vi "Main.vi"(8 "error in":errorcluster, 11 "Head Worker in":refnum<class "Head Worker.lvclass">) -> (0 "error out":errorcluster, 3 "Head Worker out":refnum<class "Head Worker.lvclass">)   [LabVIEW 2017, in "Head Worker.lvclass"]
doc: "The <b>Queued Message Handler</b> of the Worker that owns this VI."
uses:
  Head Worker.lvclass
  Head Worker.lvclass/Head Worker.ctl
  Initialization Data.ctl
  Response Cases.ctl
  Main UI/Main UI.lvclass
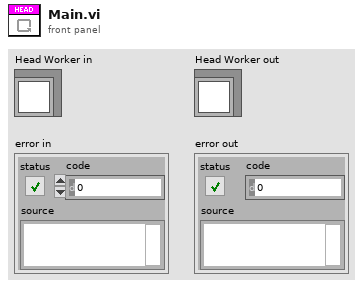
[diagram p1: front panel]
types:
  T1 = typedef "Head Worker.lvclass/Initialization Data.ctl" = cluster{"Response Cases":T2}
  T2 = typedef "Head Worker.lvclass/Response Cases.ctl" = cluster{"Placeholder - Can be deleted":string}
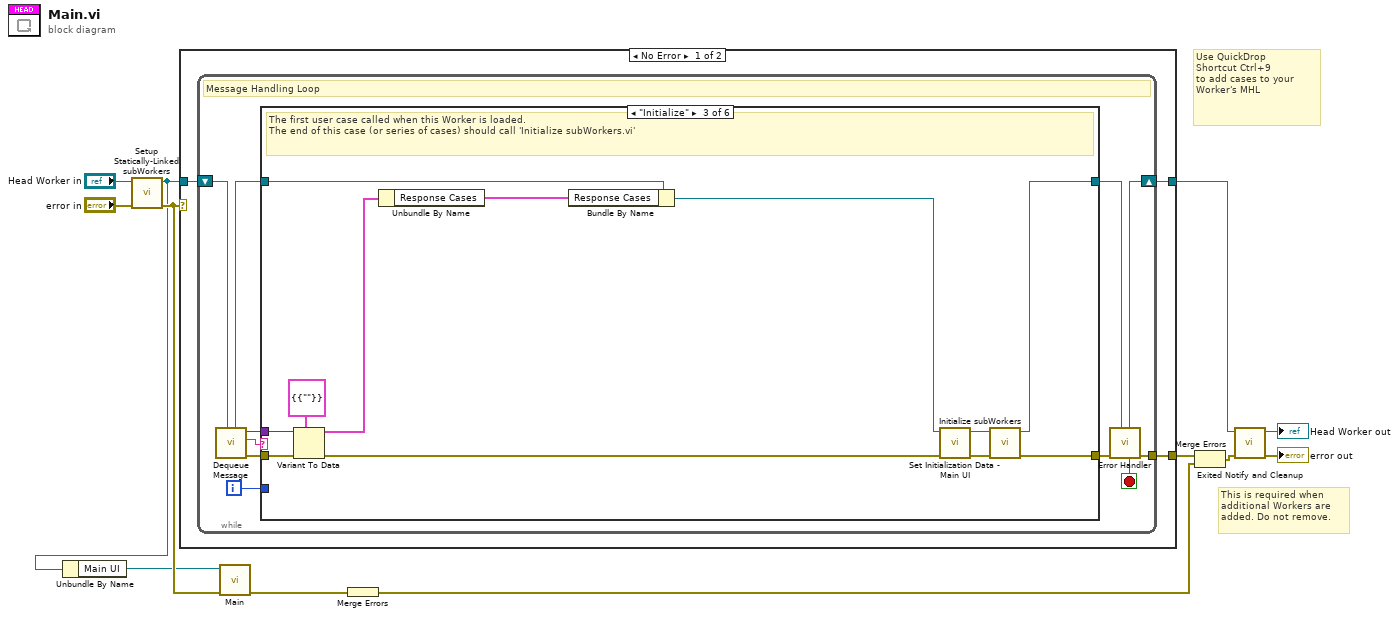
[diagram p0: block diagram]
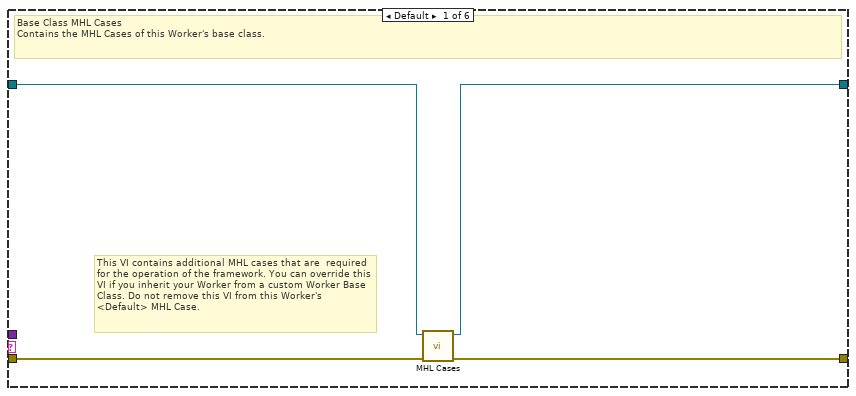
[diagram p2: hidden frame]
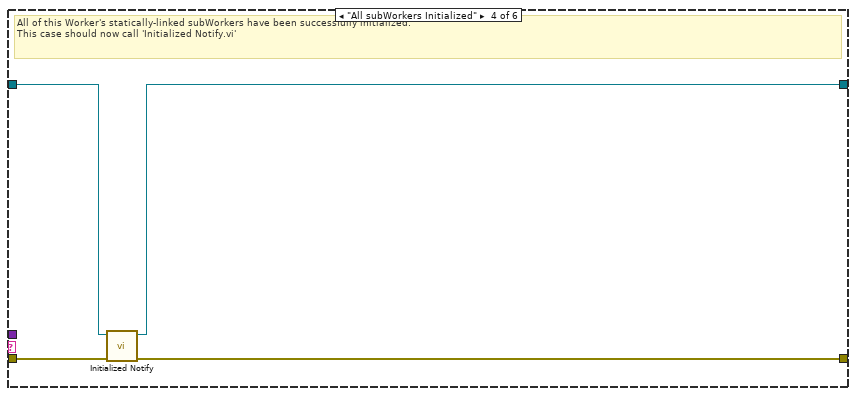
[diagram p4: hidden frame]
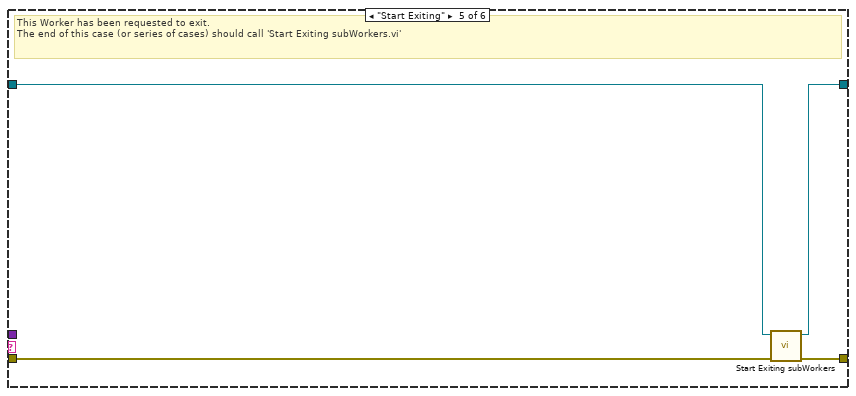
[diagram p5: hidden frame]
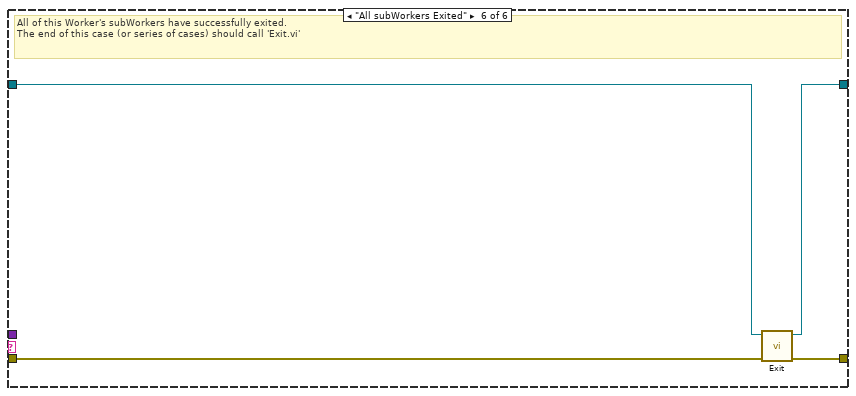
[diagram p6: hidden frame]
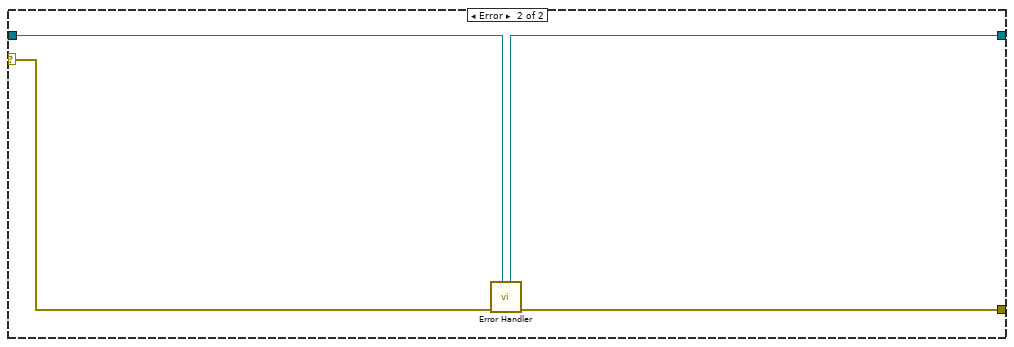
[diagram p7: hidden frame]
diagram:
  # "Use QuickDrop\nShortcut Ctrl+9\nto add cases to your\nWorker's MHL"
  # "This is required when additional Workers are added. Do not remove."
  n1 = call "Setup Statically-Linked subWorkers.vi"("error in"="error in", "Head Worker in"="Head Worker in") -> ("error out"=w6:errorcluster, "Head Worker out"=w4:refnum<class "Head Worker.lvclass">)  [unwired: 8 in]
  n2 = Unbundle By Name(w4) -> ("Main UI"=w1:refnum<class "Main UI.lvclass">)
  n3 = case shown="No Error" w6 {
    tunnel: w4 -> [w13 w58]
    tunnel: [w15 w59] -> w11
    tunnel: [w14 w57] -> w12
    selector: w6 -> [_ w60]
    frame No Error {
      n4 = while {
        shift-right: [w24] -> w14
        shift-left: w13 -> [w26]
        tunnel: [w25] -> w15
        i -> [w16]
        stop <- w17 stop-if-true
        # "Message Handling Loop"
        n5 = call-dynamic "Dequeue Message.vi"("Worker"=w26) -> ("error out"=w23:errorcluster, "Case out"=w18:string, "Data out"=w19:variant, "Worker out"=w21:refnum<class "Head Worker.lvclass">)  [unwired: 6 in, 1 out]
        n6 = case "Worker MHL Case Structure (DO NOT CHANGE LABEL NAME)" shown="\"Initialize\"" w18 {
          tunnel: w23 -> [w30 w31 w42 w48 w49 w56]
          tunnel: [w29 w31 w44 w47 w52 w55] -> w22
          tunnel: w21 -> [w28 w32 w41 w46 w50 w54]
          tunnel: [w27 w32 w43 w45 w51 w53] -> w20
          tunnel: w19 -> [_ _ w39 _ _ _]
          tunnel: w16 -> [_ _ _ _ _ _]
          frame Default {
            # "This VI contains additional MHL cases that are  required for the operation of the framework. You can override this VI if you inherit your Worker from a custom Worker Base Class. Do not remove this VI from this Worker's <Default> MHL Case."
            # "Base Class MHL Cases\nContains the MHL Cases of this Worker's base class."
            n7 = call-dynamic "MHL Cases.vi"("error in"=w30, "Worker in"=w28) -> ("error out"=w29:errorcluster, "Worker out"=w27:refnum<class "Head Worker.lvclass">)  [unwired: 8 in]
          }
          frame "------------ FRAMEWORK CASES -----------" {
            # "Start of Workers Framework Cases"
          }
          frame "Initialize" {
            # "The first user case called when this Worker is loaded.\nThe end of this case (or series of cases) should call 'Initialize subWorkers.vi'"
            n8 = Variant To Data(error in=w42, type=T1 {"Response Cases"={"Placeholder - Can be deleted"=""}} ("Cluster"), Variant=w39) -> (data=w38:T1, error out=w40:errorcluster)
            n9 = Unbundle By Name(w38) -> ("Response Cases"=w37:T2)
            n10 = Bundle By Name(cluster=w41, "Response Cases"=w37) -> (w33:refnum<class "Head Worker.lvclass">)
            n11 = call "Set Initialization Data - Main UI.vi"("error in"=w40, "Head Worker in"=w33) -> ("error out"=w35:errorcluster, "Head Worker out"=w34:refnum<class "Head Worker.lvclass">)  [unwired: 8 in]
            n12 = call-dynamic "Initialize subWorkers.vi"("error in"=w35, "Worker"=w34) -> ("error out"=w44:errorcluster, "dup Worker out"=w43:refnum<class "Head Worker.lvclass">)  [unwired: 8 in]
          }
          frame "All subWorkers Initialized" {
            # "All of this Worker's statically-linked subWorkers have been successfully initialized.\nThis case should now call 'Initialized Notify.vi'"
            n13 = call-dynamic "Initialized Notify.vi"("error in"=w48, "Worker"=w46) -> ("error out"=w47:errorcluster, "dup Worker out"=w45:refnum<class "Head Worker.lvclass">)  [unwired: 8 in]
          }
          frame "Start Exiting" {
            # "This Worker has been requested to exit. \nThe end of this case (or series of cases) should call 'Start Exiting subWorkers.vi'"
            n14 = call-dynamic "Start Exiting subWorkers.vi"("error_in"=w49, "Worker"=w50) -> ("error out"=w52:errorcluster, "dup Worker out"=w51:refnum<class "Head Worker.lvclass">)  [unwired: 8 in]
          }
          frame "All subWorkers Exited" {
            # "All of this Worker's subWorkers have successfully exited. \nThe end of this case (or series of cases) should call 'Exit.vi'"
            n15 = call-dynamic "Exit.vi"("error_in"=w56, "Worker"=w54) -> ("error out"=w55:errorcluster, "dup Worker out"=w53:refnum<class "Head Worker.lvclass">)  [unwired: 8 in]
          }
        }
        n16 = call-dynamic "Error Handler.vi"("Worker"=w20, "error_in"=w22) -> ("error out"=w25:errorcluster, "Stop Loop"=w17:bool, "Worker out"=w24:refnum<class "Head Worker.lvclass">)  [unwired: 7 in]
      }
    }
    frame Error {
      n17 = call-dynamic "Error Handler.vi"("Worker"=w58, "error_in"=w60) -> ("error out"=w59:errorcluster, "Worker out"=w57:refnum<class "Head Worker.lvclass">)  [unwired: 7 in, 1 out]
    }
  }
  n18 = call-dynamic "Main.vi"("error in"=w6, "Main UI in"=w1) -> ("error out"=w3:errorcluster)  [unwired: 8 in, 1 out]
  n19 = Merge Errors(w3) -> (w2:errorcluster)
  n20 = Merge Errors(w11, w2) -> (w8:errorcluster)
  n21 = call-dynamic "Exited Notify and Cleanup.vi"("error_in"=w8, "Worker"=w12) -> ("error out"=→"error out":errorcluster, "dup Worker out"=→"Head Worker out":refnum<class "Head Worker.lvclass">)  [unwired: 8 in]
